vi "Construct.vi"(8 "error in (no error)":errorcluster, 11 "ListenerPort":u16) -> (0 "error out":errorcluster, 3 "ServiceManager-Comms out":refnum<class "ServiceManager-Comms.lvclass">)   [LabVIEW 2020, in "ServiceManager.lvlib" / "ServiceManager-Comms.lvclass"]
uses:
  ServiceManager-Comms.lvclass
  ServiceManager-Comms.lvclass/ServiceManager-Comms.ctl
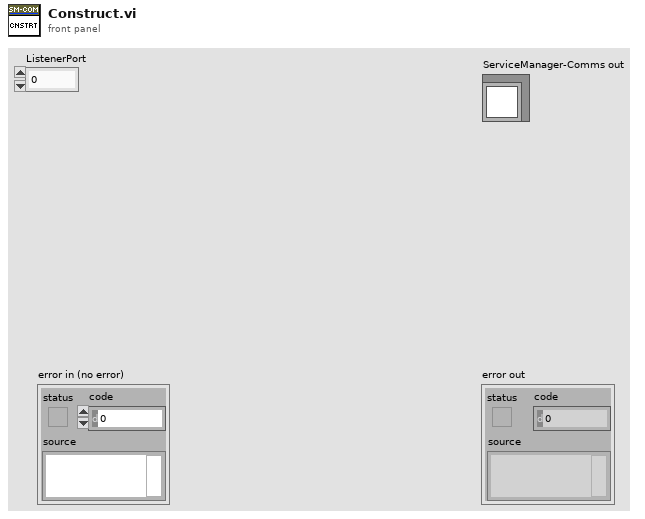
[diagram p1: front panel]
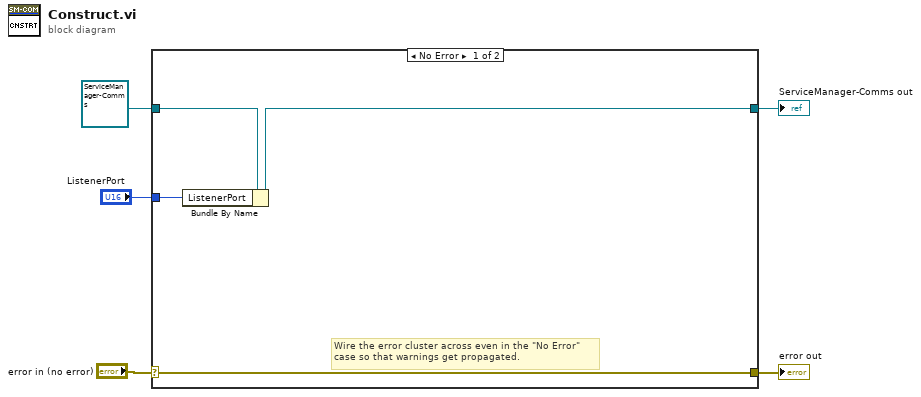
[diagram p0: block diagram]
diagram:
  n1 = case shown="No Error" "error in (no error)" {
    selector: "error in (no error)" -> [w8 w11]
    tunnel: [w8 w11] -> w4
    tunnel: [w7 w10] -> w2
    tunnel: refnum<class "ServiceManager-Comms.lvclass"> refnum ("ServiceManager-Comms in") -> [w9 w10]
    tunnel: "ListenerPort" -> [w6 _]
    frame No Error {
      # "Wire the error cluster across even in the \"No Error\"\ncase so that warnings get propagated."
      n2 = Bundle By Name(cluster=w9, "ListenerPort"=w6) -> (w7:refnum<class "ServiceManager-Comms.lvclass">)
    }
    frame Error {
    }
  }
  "error out" <- w4
  "ServiceManager-Comms out" <- w2
